vi "Alazar_SetTriggerDelay.vi"(10 "Delay in Pts":u32, 11 "DeviceIn":i32) -> (0 "Return Code":u32, 3 "DeviceOut":i32)   [LabVIEW 2022 SP3]
doc: "_____AlazarTech, Scope_____\n\nSet the Trigger delay"
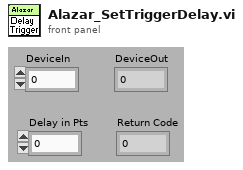
[diagram p1: front panel]
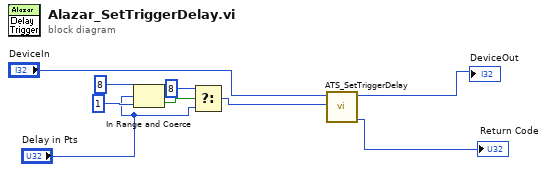
[diagram p0: block diagram]
diagram:
  n1 = In Range and Coerce(upper limit=u32 8, x="Delay in Pts", lower limit=u32 1) -> (In Range?=w9:bool)  [unwired: 1 out]
  n2 = Select(t=u32 8, s=w9, f="Delay in Pts") -> (s? t:f=w6:u32)
  n3 = call "ATS_SetTriggerDelay.vi"("Delay"=w6, "DeviceIn"="DeviceIn") -> ("Return Code"=→"Return Code":u32, "DeviceOut"=→"DeviceOut":i32)  [unwired: 8 in]
